vi "Add Channels.vi"(8 "error in (no error)":errorcluster, 10 "Channel Config":T1, 11 "Parent Ref in":T3 format="%.0x") -> (0 "error out":errorcluster)   [LabVIEW 2021, in "Software Multi-Plex System Explorer.lvlib"]
uses:
  Software Multi-Plex System Explorer.lvlib
  <vilib>/NI VeriStand/Custom Device API/Custom Device Item Ref.ctl
  Types/Channel Config.ctl
  Types/Index Type.ctl
  <vilib>/NI VeriStand/Custom Device API/Custom Device Channel.ctl
  <vilib>/NI VeriStand/Custom Device API/Custom Device Channel Type.ctl
  Shared/Constants.vi
  <vilib>/NI VeriStand/Custom Device Tools/Custom Device Utility Library/NI VeriStand - Search for All Items by GUID.vi
  <vilib>/NI VeriStand/Custom Device API/Custom Device API.lvlib
  Shared/Software Multi-Plex Shared.lvlib
  <vilib>/NI VeriStand/Custom Device Tools/Custom Device Utility Library/Custom Device Utility Library.lvlib
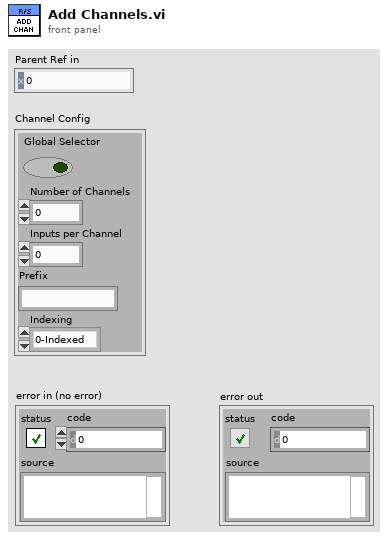
[diagram p1: front panel]
types:
  T1 = typedef "Software Multi-Plex System Explorer.lvlib/Channel Config.ctl" = cluster{"Global Selector":bool, "Number of Channels":i32, "Inputs per Channel":i32, "Prefix":string, "Indexing":T2}
  T2 = typedef "Software Multi-Plex System Explorer.lvlib/Index Type.ctl" = enum16{"0-Indexed", "1-Indexed"}
  T3 = typedef "Custom Device API.lvlib/Custom Device Item Ref.ctl" = u64
  T4 = typedef "Custom Device API.lvlib/Custom Device Channel.ctl" = cluster{"Type":T5, "Units":string, "Default Value":dbl, "Faultable":bool, "Scalable":bool}
  T5 = typedef "Custom Device API.lvlib/Custom Device Channel Type.ctl" = enum16{"Input", "Output"}
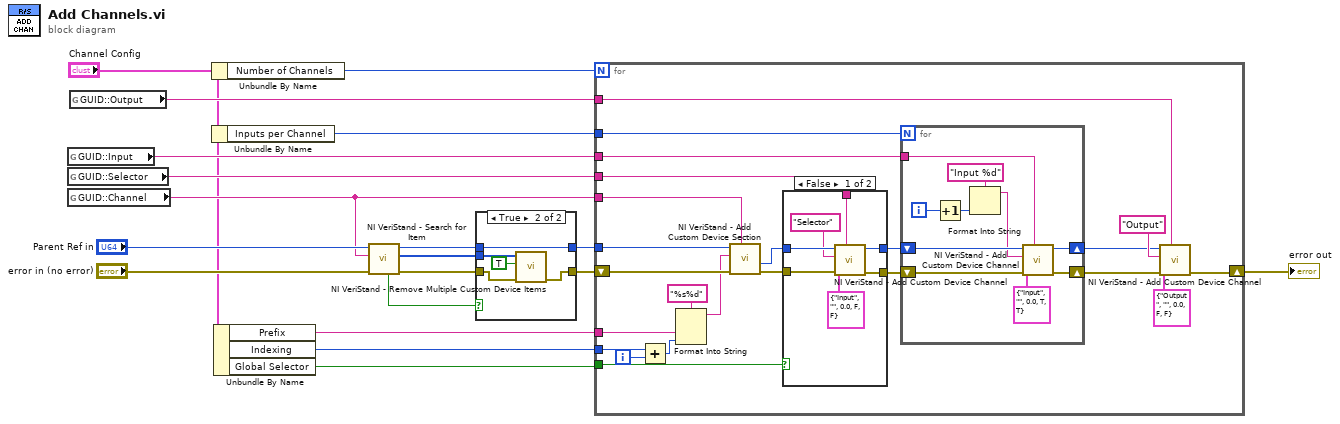
[diagram p0: block diagram]
diagram:
  n1 = global read "Constants.vi" "GUID::Input"() -> (w8:string)
  n2 = global read "Constants.vi" "GUID::Selector"() -> (w9:string)
  n3 = global read "Constants.vi" "GUID::Channel"() -> (w10:string)
  n4 = global read "Constants.vi" "GUID::Output"() -> (w7:string)
  n5 = Unbundle By Name("Channel Config") -> ("Number of Channels"=w6:i32)
  n6 = Unbundle By Name("Channel Config") -> ("Inputs per Channel"=w5:i32)
  n7 = Unbundle By Name("Channel Config") -> ("Prefix"=w1:string, "Indexing"=w2:T2, "Global Selector"=w3:bool)
  n8 = call-poly <vilib>:"NI VeriStand - Search for Item.vi"("error in"="error in (no error)", "Item GUID"=w10, "Section Ref in"="Parent Ref in") -> ("error out"=w15:errorcluster, "Item Refs"=w14:T3[], "Section Ref out"=w13:T3, "Found"=w16:bool)  [unwired: 5 in]
  n9 = case shown="True" w16 {
    tunnel: w15 -> [w20 w26]
    tunnel: w14 -> [_ w25]
    tunnel: w13 -> [w21 w23]
    tunnel: [w21 w23] -> w12
    tunnel: [w20 w24] -> w11
    frame False {
    }
    frame True {
      n10 = call <vilib>:"NI VeriStand - Remove Multiple Custom Device Items.vi"("error in (no error)"=w26, "Force Delete (F)"=TRUE, "Item Refs in"=w25) -> ("error out"=w24:errorcluster)  [unwired: 7 in, 1 out]
    }
  }
  n11 = for {
    N: w6 -> [_]
    tunnel: w12 -> [w33]
    shift-right: [w43] -> w19
    shift-left: w11 -> [w34]
    tunnel: w10 -> [w40]
    tunnel: w5 -> [w38]
    tunnel: w9 -> [w39]
    tunnel: w8 -> [w37]
    tunnel: w7 -> [w36]
    tunnel: w3 -> [w35]
    tunnel: w2 -> [w28]
    tunnel: w1 -> [w30]
    i -> [w27]
    n12 = Add(x=w28, y=w27) -> (x+y=w29:i32)
    n13 = Format Into String(format string="%s%d", w30, w29) -> (resulting string=w31:string)  [unwired: 2 in, 1 out]
    n14 = call <vilib>:"NI VeriStand - Add Custom Device Section.vi"("GUID (Default Section)"=w40, "error in (no error)"=w34, "Section Name"=w31, "Parent Ref in"=w33) -> ("error out"=w49:errorcluster, "Section Ptr"=w48:T3)  [unwired: 4 in, 2 out]
    n15 = case shown="False" w35 {
      tunnel: w49 -> [w56 w58]
      tunnel: w48 -> [w55 w57]
      tunnel: [w52 w58] -> w47
      tunnel: [w51 w57] -> w46
      tunnel: w39 -> [w50 _]
      frame False {
        n16 = call <vilib>:"NI VeriStand - Add Custom Device Channel.vi"("GUID (Default Channel)"=w50, "error in (no error)"=w56, "Channel"=T4 {"Type"=enum."Input", "Units"="", "Default Value"=0.0, "Faultable"=FALSE, "Scalable"=FALSE}, "Channel Name"="Selector", "Parent Ref in"=w55) -> ("error out"=w52:errorcluster, "Parent Ref out"=w51:T3)  [unwired: 3 in, 2 out]
      }
      frame True {
      }
    }
    n17 = for {
      N: w38 -> [_]
      shift-right: [w65] -> w42
      shift-left: w47 -> [w68]
      shift-right: [w64] -> w41
      shift-left: w46 -> [w67]
      tunnel: w37 -> [w63]
      i -> [w60]
      n18 = Increment(x=w60) -> (x+1=w61:i32)
      n19 = Format Into String(format string="Input %d" ("Channel Name"), w61) -> (resulting string=w59:string)  [unwired: 2 in, 1 out]
      n20 = call <vilib>:"NI VeriStand - Add Custom Device Channel.vi"("GUID (Default Channel)"=w63, "error in (no error)"=w68, "Channel"=T4 {"Type"=enum."Input", "Units"="", "Default Value"=0.0, "Faultable"=TRUE, "Scalable"=TRUE}, "Channel Name"=w59, "Parent Ref in"=w67) -> ("error out"=w65:errorcluster, "Parent Ref out"=w64:T3)  [unwired: 3 in, 2 out]
    }
    n21 = call <vilib>:"NI VeriStand - Add Custom Device Channel.vi"("GUID (Default Channel)"=w36, "error in (no error)"=w42, "Channel"=T4 {"Type"=enum."Output", "Units"="", "Default Value"=0.0, "Faultable"=FALSE, "Scalable"=FALSE}, "Channel Name"="Output", "Parent Ref in"=w41) -> ("error out"=w43:errorcluster)  [unwired: 3 in, 3 out]
  }
  "error out" <- w19
